vi "installer_create_file.vi"(4 "special_file":path, 6 "distribution_folder":path, 8 "error in (no error)":errorcluster, 11 "build_specifications":T1) -> (0 "error out":errorcluster)   [LabVIEW 2015, in "lv-builder.lvlib"]
uses:
  lv-builder.lvlib
  lv-build/public/_controls/build_specification.ctl
  lv-build/public/_controls/build_type.ctl
  <userlib>/antonio-alexander/lv-bin-7zip/public/api/v1/_controls/config_include.ctl
  <userlib>/antonio-alexander/lv-bin-7zip/public/api/v1/_controls/config_value.ctl
  <userlib>/antonio-alexander/lv-bin-7zip/public/api/v1/advanced/make_installer_exe_custom.vi
  <userlib>/antonio-alexander/lv-bin-7zip/public/api/v1/v1.lvlib
  lv-build/lv-build.lvlib
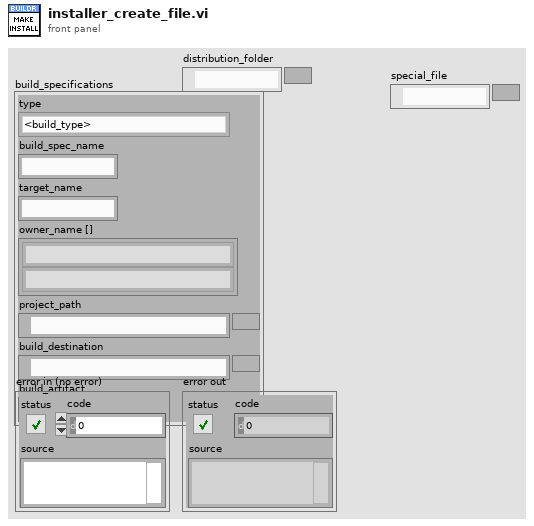
[diagram p1: front panel]
types:
  T1 = typedef "lv-build.lvlib/build_specification.ctl" = cluster{"type":T2, "build_spec_name":string, "target_name":string, "owner_name []":string[], "project_path":path, "build_destination":path, "build_artifact":path}
  T2 = typedef "lv-build.lvlib/build_type.ctl" = enum16{"<build_type>", "application_pc", "application_rt", "installer", "llb", "lvlibp", "zip", "fpga", "<null>"}
  T3 = typedef "lv-bin-7zip.lvlib/v1.lvlib/config_value.ctl" = cluster{"title":string, "begin_prompt":string, "run_program":string, "directory":string, "execute_file":string, "execute_parameters":string, "progress":bool}
  T4 = typedef "lv-bin-7zip.lvlib/v1.lvlib/config_include.ctl" = cluster{"title":bool, "begin_prompt":bool, "progress":bool, "run_program":bool, "directory":bool, "execute_file":bool, "execute_parameters":bool}
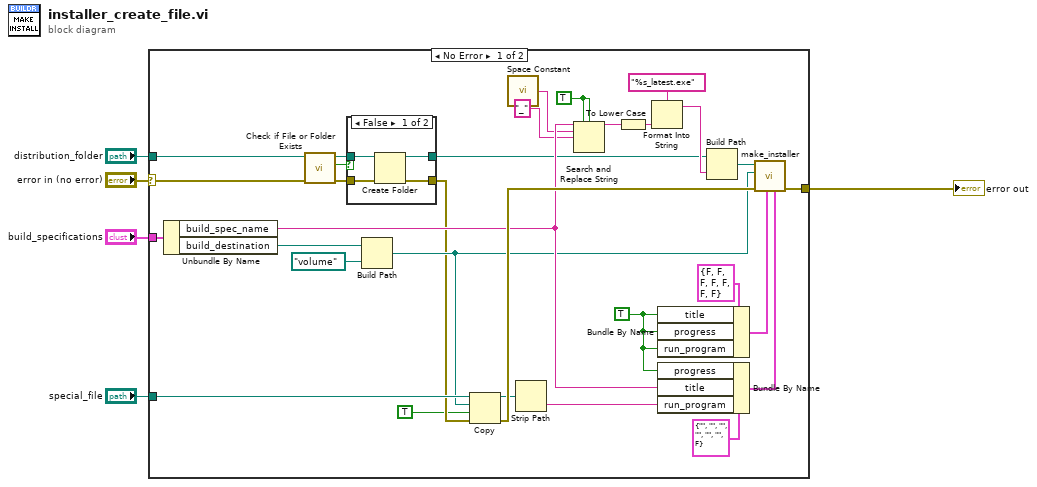
[diagram p0: block diagram]
diagram:
  n1 = case shown="No Error" "error in (no error)" {
    selector: "error in (no error)" -> [w19 w43]
    tunnel: "build_specifications" -> [w35 _]
    tunnel: [w31 w43] -> w5
    tunnel: "special_file" -> [w12 _]
    tunnel: "distribution_folder" -> [w6 _]
    frame No Error {
      w25 = TRUE ("replace all? (F)")
      w13 = TRUE ("title")
      n2 = Unbundle By Name(w35) -> ("build_spec_name"=w23:string, "build_destination"=w30:path)
      n3 = call <vilib>:"Check if File or Folder Exists.vi"("error in (no error)"=w19, "path"=w6) -> ("error out"=w18:errorcluster, "file or folder exists?"=w15:bool, "dup path"=w17:path)  [unwired: 7 in]
      n4 = case shown="False" w15 {
        tunnel: w18 -> [w40 w41]
        tunnel: w17 -> [w39 w42]
        tunnel: [w38 w42] -> w16
        tunnel: [w37 w41] -> w10
        frame False {
          n5 = Create Folder(path (use dialog)=w39, error in=w40) -> (created path=w38:path, error out=w37:errorcluster)  [unwired: 1 in, 1 out]
        }
        frame True {
        }
      }
      n6 = Build Path(base path=w30, name or relative path=path "volume") -> (appended path=w11:path)
      n7 = Copy(8:w10, 9:TRUE ("overwrite (F)"), 10:w11, 11:w12) -> (0:w36:errorcluster, 3:w9:path)  [unwired: 1 in, 1 out]
      n8 = call <vilib>:"Space Constant.vi"() -> ("String"=w21:string)
      n9 = Strip Path(path=w9) -> (name=w8:string)  [unwired: 1 out]
      n10 = Search and Replace String(replace all?=w25, case sensitive?=w25, input string=w23, search string=w21, replace string="_" ("search string")) -> (result string=w22:string)  [unwired: 3 in, 3 out]
      n11 = To Lower Case(string=w22) -> (all lower case string=w24:string)
      n12 = Format Into String(format string="%s_latest.exe", w24) -> (resulting string=w33:string)  [unwired: 2 in, 1 out]
      n13 = Bundle By Name(cluster=T4 {"title"=FALSE, "begin_prompt"=FALSE, "progress"=FALSE, "run_program"=FALSE, "directory"=FALSE, "execute_file"=FALSE, "execute_parameters"=FALSE} ("config_include"), "title"=w13, "progress"=w13, "run_program"=w13) -> (w27:T4)
      n14 = Bundle By Name(cluster=T3 {"title"="", "begin_prompt"="", "run_program"="", "directory"="", "execute_file"="", "execute_parameters"="", "progress"=FALSE} ("config_value"), "progress"=w13, "title"=w23, "run_program"=w8) -> (w26:T3)
      n15 = Build Path(base path=w16, name or relative path=w33) -> (appended path=w32:path)
      n16 = call-poly <userlib>:"make_installer.vi"("config_value"=w26, "config_include"=w27, "error in (no error)"=w36, "installer_directory"=w11, "setup_filename in"=w32) -> ("error out"=w31:errorcluster)  [unwired: 5 in, 1 out]
    }
    frame Error {
    }
  }
  "error out" <- w5
